vi "Verify Vcc AC RMS.vi"(8 "error in":errorcluster, 11 "Delay Time (s)":dbl=5.0) -> (0 "error out":errorcluster, 2 "Ch Values":dbl[](array[numeric]), 3 "return type":i32)   [LabVIEW 2015]
doc: "This VI will set the DAQ analog output channel to generate a Sine Wave, 62.5Hz, 50% duty cycle, 5Vpeak, 2.5Vdc offset, and use dll function \"ReadAcRmsChanValues to read an AC RMS reading on Channels 1 & 2. Calibration values are also returned to properly calculate the final result. Note that the scale is locked to 5 Volts. This function is intended to be used with the pre-defined AC RMS Test reading from the Mfg. Test specification."
uses:
  ScannerDiagDLL.dll
panel:
  out "pnChan2SpanOffset":i32
  out "pnChan2ZeroOffset":i32
  out "pnChan2Value":i32
  out "pnChan1SpanOffset":i32
  out "pnChan1ZeroOffset":i32
  out "pnChan1Value":i32
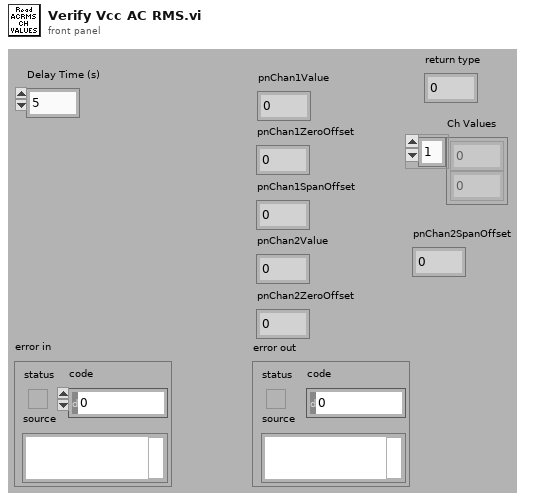
[diagram p1: front panel]
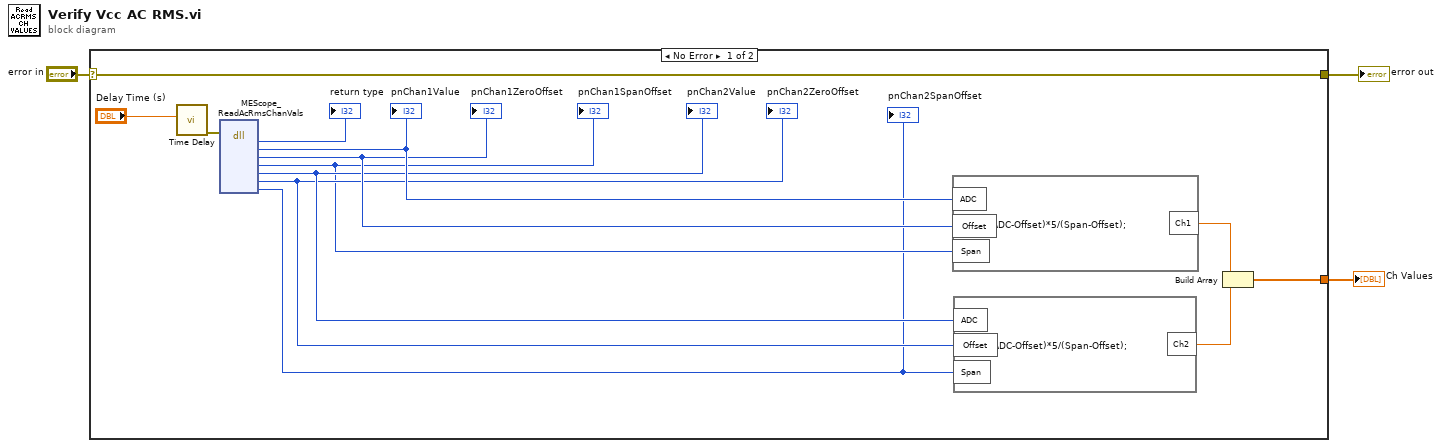
[diagram p0: block diagram]
diagram:
  n1 = case shown="No Error" "error in" {
    selector: "error in" -> [w8 w17]
    tunnel: [w8 w17] -> w2
    tunnel: [w4 _] -> w1
    frame No Error {
      n2 = call "Time Delay"("Delay Time (s)"="Delay Time (s)") -> ("error out"=w15:errorcluster)  [unwired: 10 in]
      n3 = dll-call lib="C:/ModisEdge/TabletScope/Test Sequence/Code Modules/DLL/ScannerDiagDLL.dll" fn="MEScope_ReadAcRmsChanVals"(error in=w15) -> ("return type"=→"return type":i32, "pnChan1Value"=w13:i32, "pnChan1ZeroOffset"=w12:i32, "pnChan1SpanOffset"=w9:i32, "pnChan2Value"=w11:i32, "pnChan2ZeroOffset"=w10:i32, "pnChan2SpanOffset"=w5:i32)  [unwired: 8 in, 2 out]
      "pnChan1Value" <- w13
      "pnChan1ZeroOffset" <- w12
      "pnChan1SpanOffset" <- w9
      "pnChan2Value" <- w11
      "pnChan2ZeroOffset" <- w10
      "pnChan2SpanOffset" <- w5
      n4 = formula code="Ch1=(ADC-Offset)*5/(Span-Offset);"("ADC"=w13, "Offset"=w12, "Span"=w9) -> ("Ch1"=w7:dbl)
      n5 = formula code="Ch2=(ADC-Offset)*5/(Span-Offset);"("ADC"=w11, "Offset"=w10, "Span"=w5) -> ("Ch2"=w6:dbl)
      n6 = Build Array(w7, w6) -> (w4:dbl[])
    }
    frame Error {
    }
  }
  "error out" <- w2
  "Ch Values" <- w1
